vi "Insert Ramp Time Step.vi"(0 "VISA resource name":refnum<visa-resource-name>, 1 "Unit Address (1)":i16=1, 2 "Channel 1 Guarantee Soak (F: Off)":bool, 3 "Channel 2 Guarantee Soak (F: Off)":bool, 5 "Time (0; 0; 1)":i16[](array[numeric])=[0, 0, 1], 7 "Set Point Channel 1 (75.0)":dbl=75.0 format="%.2f", 9 "Set Point Channel 2 (75.0)":dbl=75.0 format="%.2f", 11 "error in (no error)":errorcluster {"code" format="%.0x"}, 12 "Channel 1 PID Set (1)":u16=1, 13 "Channel 2 PID Set (6)":u16=6) -> (4 "VISA resource name out":refnum<visa-resource-name>, 15 "error out":errorcluster {"code" format="%.0x"})   [LabVIEW 2010]
doc: "This is second part of two VIs, that inserts Ramp Time Step. This VI sets set point, PID set, time and guarantee soak.\n\nNote: For correct function VIs MUST be activated in this sequence:\n1. WLF4 Insert Ramp Time Step Event.vi\n2. WLF4 Insert Ramp Time Step.vi"
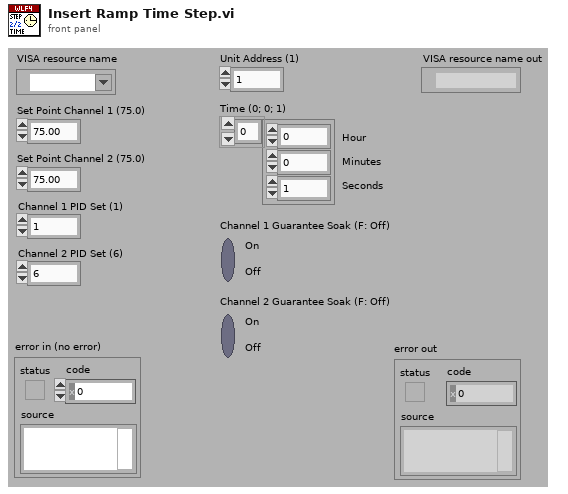
[diagram p1: front panel]
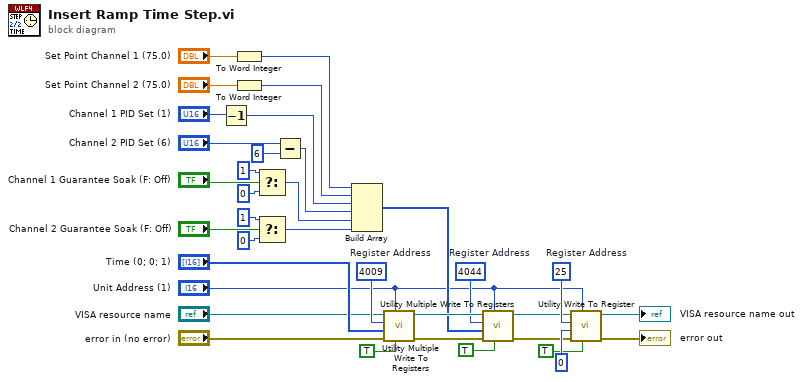
[diagram p0: block diagram]
diagram:
  w19 = u16 4044  # Register Address
  w22 = u16 4009  # Register Address
  w29 = u16 25  # Register Address
  n1 = Decrement(x="Channel 1 PID Set (1)") -> (x-1=w10:u16)
  n2 = To Word Integer(number="Set Point Channel 1 (75.0)") -> (16bit integer=w15:i16)
  n3 = To Word Integer(number="Set Point Channel 2 (75.0)") -> (16bit integer=w16:i16)
  n4 = Select(t=1, s="Channel 1 Guarantee Soak (F: Off)", f=0) -> (s? t:f=w17:i32)
  n5 = Select(t=1, s="Channel 2 Guarantee Soak (F: Off)", f=0) -> (s? t:f=w18:i32)
  n6 = Subtract(x="Channel 2 PID Set (6)", y=u16 6) -> (x-y=w8:u16)
  n7 = Build Array(w15, w16, w10, w8, w17, w18) -> (w14:i32[])
  n8 = call "Utility Multiple Write To Registers.vi"("Direct Action?"=TRUE, "Unit Address (1)"="Unit Address (1)", "error in (no error)"="error in (no error)", "Array Of Data"="Time (0; 0; 1)", "Register Address (0)"=w22, "VISA resource name"="VISA resource name") -> ("error out"=w20:errorcluster, "VISA resource name out"=w21:refnum<visa-resource-name>)  [unwired: 4 in]
  n9 = call "Utility Multiple Write To Registers.vi"("Direct Action?"=TRUE, "Unit Address (1)"="Unit Address (1)", "error in (no error)"=w20, "Array Of Data"=w14, "Register Address (0)"=w19, "VISA resource name"=w21) -> ("error out"=w12:errorcluster, "VISA resource name out"=w13:refnum<visa-resource-name>)  [unwired: 4 in]
  n10 = call "Utility Write To Register.vi"("Direct Action?"=TRUE, "Unit Address (1)"="Unit Address (1)", "error in (no error)"=w12, "Data (0)"=i16 0, "Register Address (0)"=w29, "VISA resource name"=w13) -> ("error out"=→"error out":errorcluster, "VISA resource name out"=→"VISA resource name out":refnum<visa-resource-name>)  [unwired: 4 in]
